vi "RT_HX711.vi"() -> ()   [LabVIEW 2019]
uses:
  <vilib>/FPGAPlugInAG/myRIO-1900/niLvFpga_Open_myRIO-1900.vi
  <vilib>/rvi/interface/common/dynamic/niFpgaDynamicAddResources.vi
  <vilib>/Utility/error.llb/Error Cluster From Error Code.vi
  <vilib>/rvi/errors/niLvFpgaAdjustHostInterfaceError.vi
  <vilib>/FPGAPlugInAG/Dynamic/niLvFpga_Close_Dynamic.vi
  <vilib>/rvi/interface/nirviOpenFPGA/nirviOpenFPGA.xnode
  FPGA Bitfiles/gpass2_FPGATarget_qweer_tUgOk1yh16s.lvbitx
  hx711/qweer.vi
  <vilib>/rvi/interface/nirviReadWriteControl/nirviReadWriteControl.xnode
  <vilib>/rvi/interface/nirviCloseFPGA/nirviCloseFPGA.xnode
  <vilib>/rvi/interface/Simulation/niFpgaSimulationCallBeginRW.vi
  NiFpgaLv.dll
panel:
  out "Data":i32
  in  "stop":bool
  out "Waveform Chart":i32(graph)
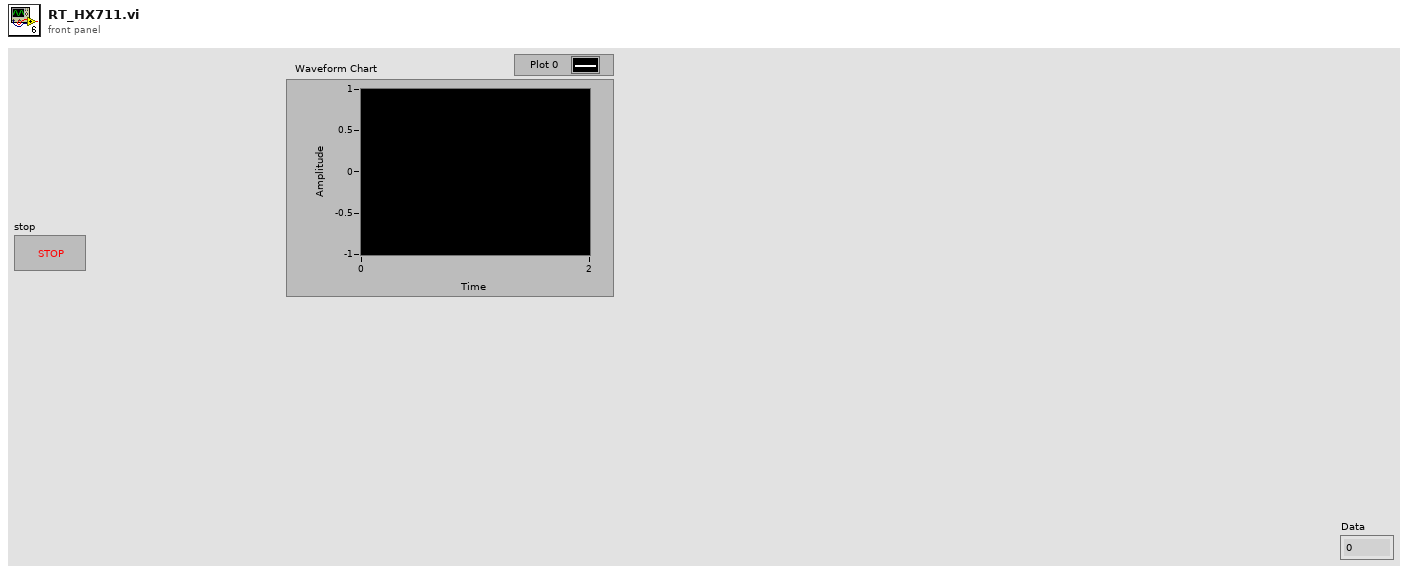
[diagram p1: front panel]
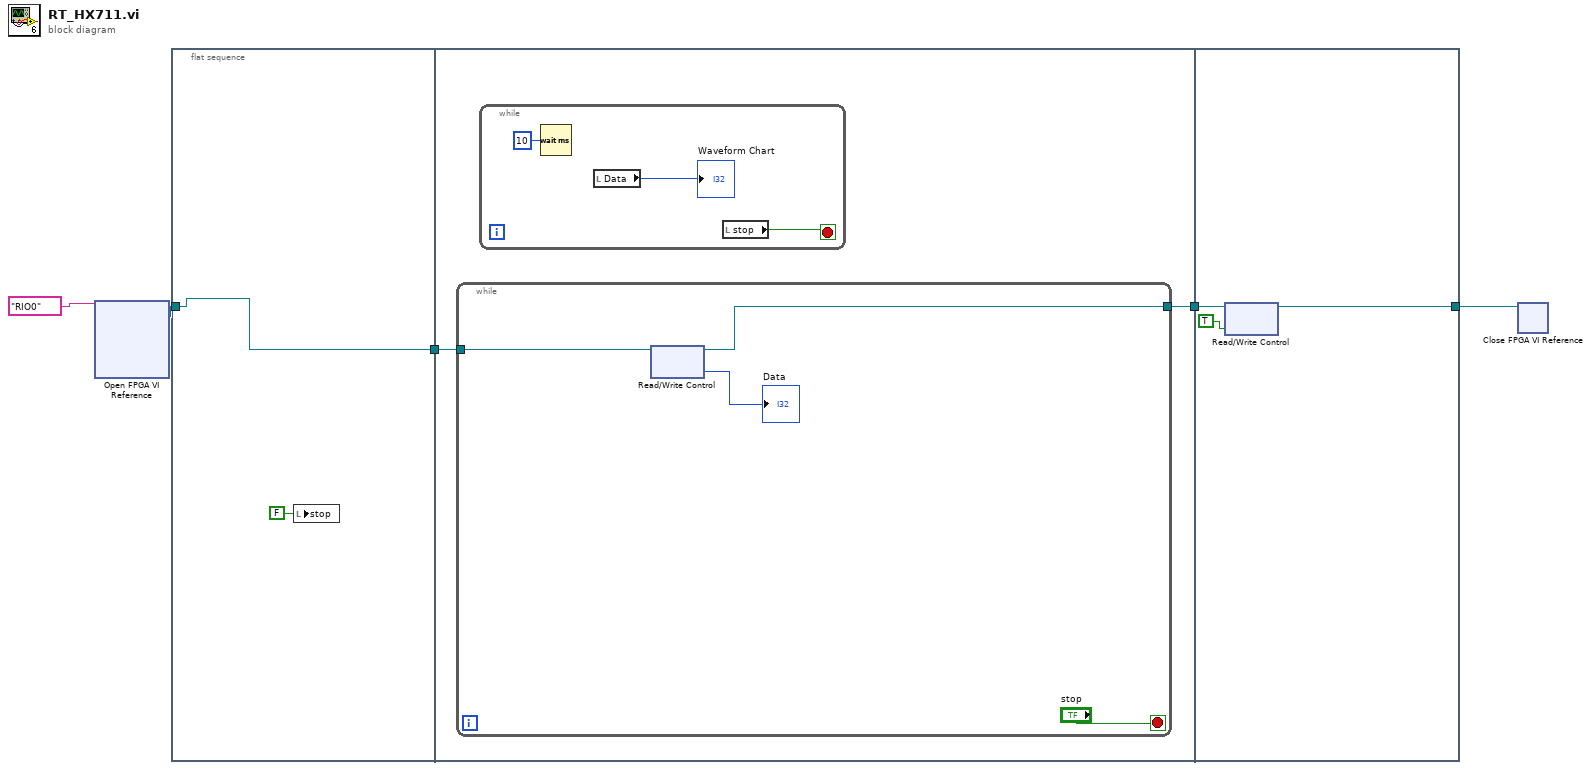
[diagram p0: block diagram]
diagram:
  n1 = xnode "Open FPGA VI Reference"("resource name"=tag "RIO0") -> ("FPGA VI Reference Out"=w3:refnum<k20>)  [unwired: 1 in, 1 out]
  n2 = flat-sequence {
    tunnel: w3 -> [w6]
    tunnel: [w6] -> w2
    tunnel: w2 -> [w9]
    tunnel: [w8] -> w1
    tunnel: [w18] -> w5
    tunnel: w1 -> [w17]
    frame #0 {
      n3 = local write "stop"(FALSE ("stop")) -> ()
    }
    frame #1 {
      n4 = while {
        tunnel: w9 -> [w15]
        tunnel: [w14] -> w8
        stop <- "stop" stop-if-true
        n5 = xnode "Read/Write Control"("FPGA VI Reference In"=w15) -> ("FPGA VI Reference Out"=w14:refnum<k20>, "Data"=→"Data":i32)  [unwired: 1 in, 1 out]
      }
      n6 = while {
        stop <- w12 stop-if-true
        n7 = Wait (ms)(milliseconds to wait=u32 10) -> ()  [unwired: 1 out]
        n8 = local read "Data"() -> (→"Waveform Chart":i32)
        n9 = local read "stop"() -> (w12:bool)
      }
    }
    frame #2 {
      n10 = xnode "Read/Write Control"("FPGA VI Reference In"=w17, "stop"=TRUE) -> ("FPGA VI Reference Out"=w18:refnum<k20>)  [unwired: 1 in, 1 out]
    }
  }
  n11 = xnode "Close FPGA VI Reference"("FPGA VI Reference In"=w5) -> ()  [unwired: 1 in, 1 out]
